vi "Send Update Task Setpoint.vi"(6 "Task Ident":string, 7 "Message Priority (Normal)":T1=enum."Normal", 8 "error in (no error)":errorcluster, 9 "Data":variant, 10 "Setpoint Ident":string, 11 "Message Enqueuer":refnum<class "Message Enqueuer.lvclass">) -> (0 "error out":errorcluster, 3 "Message Enqueuer out":refnum<class "Message Enqueuer.lvclass">)   [LabVIEW 2024, in "ISeries UI Actor.lvlib" / "Update Task Setpoint Msg.lvclass"]
doc: "This VI sends the message to an actor."
uses:
  Update Task Setpoint Msg.lvclass
  Update Task Setpoint Msg.lvclass/Update Task Setpoint Msg.ctl
  <vilib>/ActorFramework/Message Enqueuer/Message Enqueuer.lvclass
  C:/Program Files/National Instruments/LabVIEW 2024/vi.lib/ActorFramework/Message/Message.lvclass
  D:/git/HAL/MAL/Series/ISeries UI Actor/ISeries UI Actor Messages/Update Task Setpoint Msg/Update Task Setpoint Msg.lvclass
  <vilib>/ActorFramework/Message Enqueuer/Message Priority.ctl
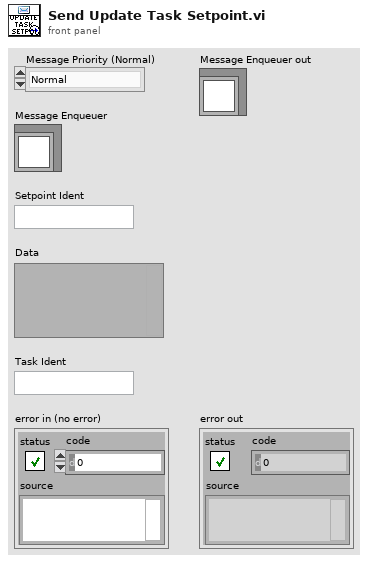
[diagram p1: front panel]
types:
  T1 = typedef "Actor Framework.lvlib/Message Enqueuer.lvclass/Message Priority.ctl" = enum16{"Low", "Normal", "High"}
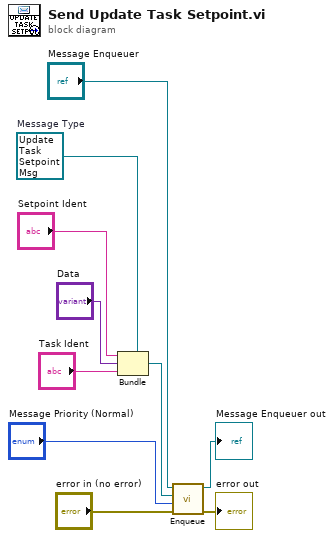
[diagram p0: block diagram]
diagram:
  w7 = refnum<class "Update Task Setpoint Msg.lvclass"> refnum  # Message Type
  n1 = Bundle(cluster=w7, "Setpoint Ident", "Data", "Task Ident") -> (w6:refnum<class "Update Task Setpoint Msg.lvclass">)
  n2 = call <vilib>:"Enqueue.vi"("error in (no error)"="error in (no error)", "Message Priority (Normal)"="Message Priority (Normal)", "Message"=w6, "Message Enqueuer in"="Message Enqueuer") -> ("error out"=→"error out":errorcluster, "Message Enqueuer in"=→"Message Enqueuer out":refnum<class "Message Enqueuer.lvclass">)  [unwired: 6 in]
